vi "reprocess orientation3.vi"(9 "use_v1_algorithm":bool, 10 "orientation_model":u32(ring) items=["APDM_ORIENTATION_MODEL_ALL", "APDM_ORIENTATION_MODEL_NO_MAG", "APDM_ORIENTATION_MODEL_UNDISTURBED_MAG"], 11 "file_in":string) -> (2 "function return":i32, 3 "file_in out":string)   [LabVIEW 2019, in "apdm.lvlib"]
doc: "APDM_EXPORT int apdm_reprocess_orientation3(char *file_in, apdm_orientation_model_t orientation_model, bool use_v1_algorithm);"
uses:
  apdm.lvlib
  Lee Lab/CP FES Walking 2018/Code/Working/LabVIEW/apdm.dll
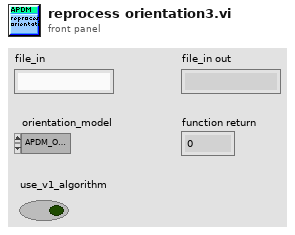
[diagram p1: front panel]
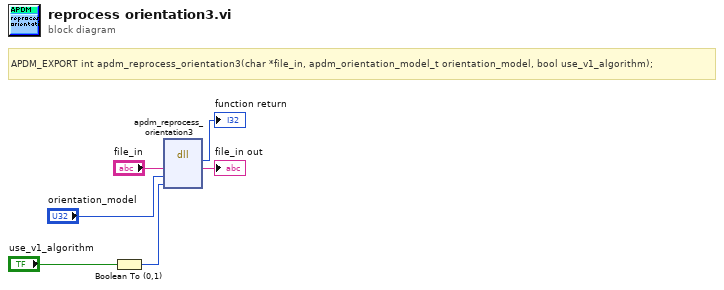
[diagram p0: block diagram]
diagram:
  # "APDM_EXPORT int apdm_reprocess_orientation3(char *file_in, apdm_orientation_model_t orientation_model, bool use_v1_algorithm);"
  n1 = Boolean To (0,1)(Boolean="use_v1_algorithm") -> (0, 1=w1:i16)
  n2 = dll-call lib="C:/Users/jfalesi/Dropbox/Lee Lab/CP FES Walking 2018/Code/Working/LabVIEW/apdm.*" fn="apdm_reprocess_orientation3"("file_in"="file_in", "orientation_model"="orientation_model", "use_v1_algorithm"=w1) -> (→"function return":i32, "file_in"=→"file_in out":string)  [unwired: 5 in, 2 out]
